vi "Queue Send Message.vi"(8 "error in (no error)":errorcluster caption="Error In", 9 "Data":variant, 10 "Message":string, 11 "Queue Name":string) -> (0 "error out":errorcluster caption="Error Out", 2 "New？":bool, 3 "Queue Out":refnum<queue>)   [LabVIEW 2020]
uses:
  Queue Message.ctl
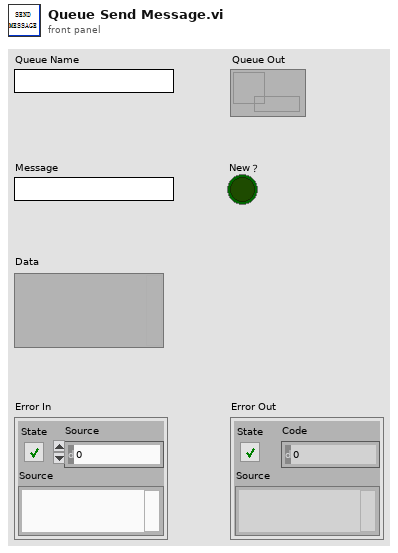
[diagram p1: front panel]
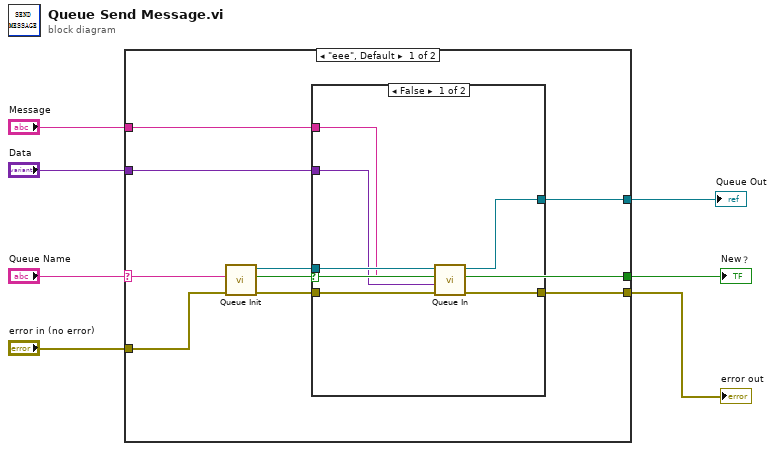
[diagram p0: block diagram]
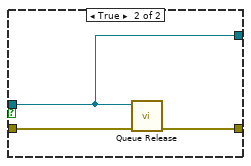
[diagram p2: hidden frame]
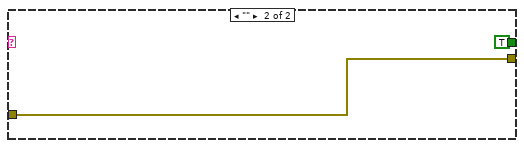
[diagram p3: hidden frame]
diagram:
  n1 = case shown="\"eee\", Default" "Queue Name" {
    selector: "Queue Name" -> [w10 _]
    tunnel: "Data" -> [w16 _]
    tunnel: [w15 w27] -> w6
    tunnel: "Message" -> [w14 _]
    tunnel: [w11 TRUE ("New?")] -> w4
    tunnel: "error in (no error)" -> [w9 w27]
    tunnel: [w8 _] -> w1
    frame "eee", Default {
      n2 = call "Queue Init.vi"("error in (no error)"=w9, "Queue Name"=w10) -> ("错误输出"=w12:errorcluster, "New?"=w11:bool, "Queue Out"=w13:refnum<queue>)  [unwired: 7 in]
      n3 = case shown="False" w11 {
        tunnel: w13 -> [w22 w23]
        tunnel: w12 -> [w21 w25]
        tunnel: w16 -> [w20 _]
        tunnel: [w19 w24] -> w15
        tunnel: w14 -> [w18 _]
        tunnel: [w17 w23] -> w8
        frame False {
          n4 = call "Queue In.vi"("error in (no error)"=w21, "Data"=w20, "Message"=w18, "Queue In"=w22) -> ("error out"=w19:errorcluster, "Queue Out"=w17:refnum<queue>)  [unwired: 6 in]
        }
        frame True {
          n5 = call "Queue Release.vi"("error in (no error)"=w25, "Queue In"=w23) -> ("error out"=w24:errorcluster)  [unwired: 9 in]
        }
      }
    }
    frame "" {
    }
  }
  "error out" <- w6
  "New？" <- w4
  "Queue Out" <- w1
